vi "ReadWrite.ReadValues.vi"(8 "error in (no error)":errorcluster, 11 "ReadWrite in":refnum<class "ReadWrite.lvclass">) -> (0 "error out":errorcluster, 2 "Values":dbl[](array[numeric]), 3 "ReadWrite out":refnum<class "ReadWrite.lvclass">)   [LabVIEW 2027, in "Data Access Engine (Express).lvlib" / "ReadWrite.lvclass"]
uses:
  ReadWrite.lvclass
  ReadWrite.lvclass/ReadWrite.ctl
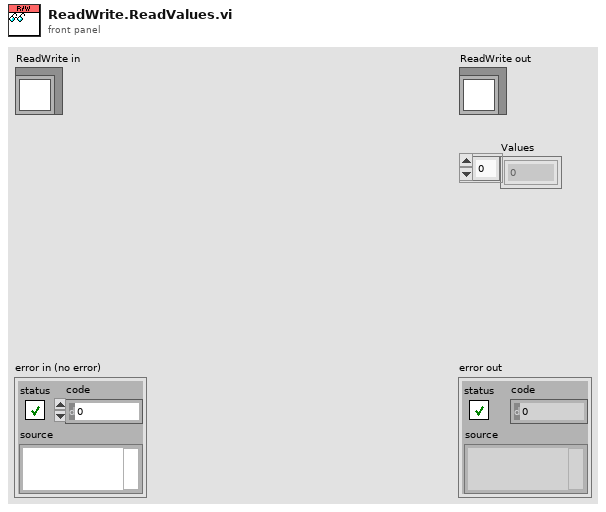
[diagram p1: front panel]
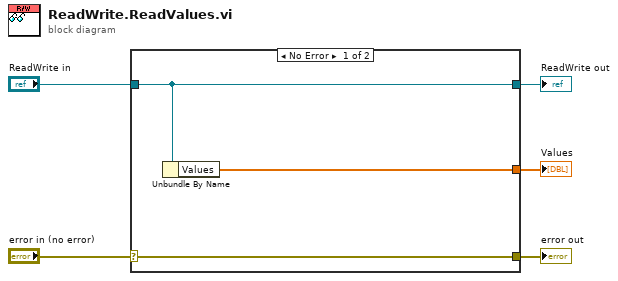
[diagram p0: block diagram]
diagram:
  n1 = case shown="No Error" "error in (no error)" {
    selector: "error in (no error)" -> [w8 w9]
    tunnel: [w8 w9] -> w4
    tunnel: [w7 w10] -> w2
    tunnel: "ReadWrite in" -> [w7 w10]
    tunnel: [w6 _] -> w1
    frame No Error {
      n2 = Unbundle By Name(w7) -> ("Values"=w6:dbl[])
    }
    frame Error {
    }
  }
  "error out" <- w4
  "ReadWrite out" <- w2
  "Values" <- w1
